vi "busy_wait_embed.vi"(4 "dialog_reference":refnum<vi>, 6 "knob_reference":refnum<vi>, 7 "caller":refnum<vi>, 8 "error in (no error)":errorcluster, 11 "configuration":T1={"dialog_text"="", "boolean_text_1"="", "boolean_text_2"="", "boolean_text_3"="", "inner_color"=16711680, "outer_color"=6618880, "wait_s"=nan, "error_status"=FALSE, "error_source"="", "error_details"="", "string []"=[], "custom_entry"=FALSE}) -> (0 "error out":errorcluster, 3 "failed/cancelled?":bool)   [LabVIEW 2015, in "lv-dialog-interfaces.lvlib"]
uses:
  lv-dialog-interfaces.lvlib
  lv-dialog/api/v1/public/_controls/configuration.ctl
  _controls/dialog_type.ctl
  _controls/hmi_references.ctl
  lv-dialog/api/v1/public/_controls/dialog_selection.ctl
  <vilib>/ptbypt/NI_PtbyPt.lvlib
  lv-dialog/api/v1/v1.lvlib
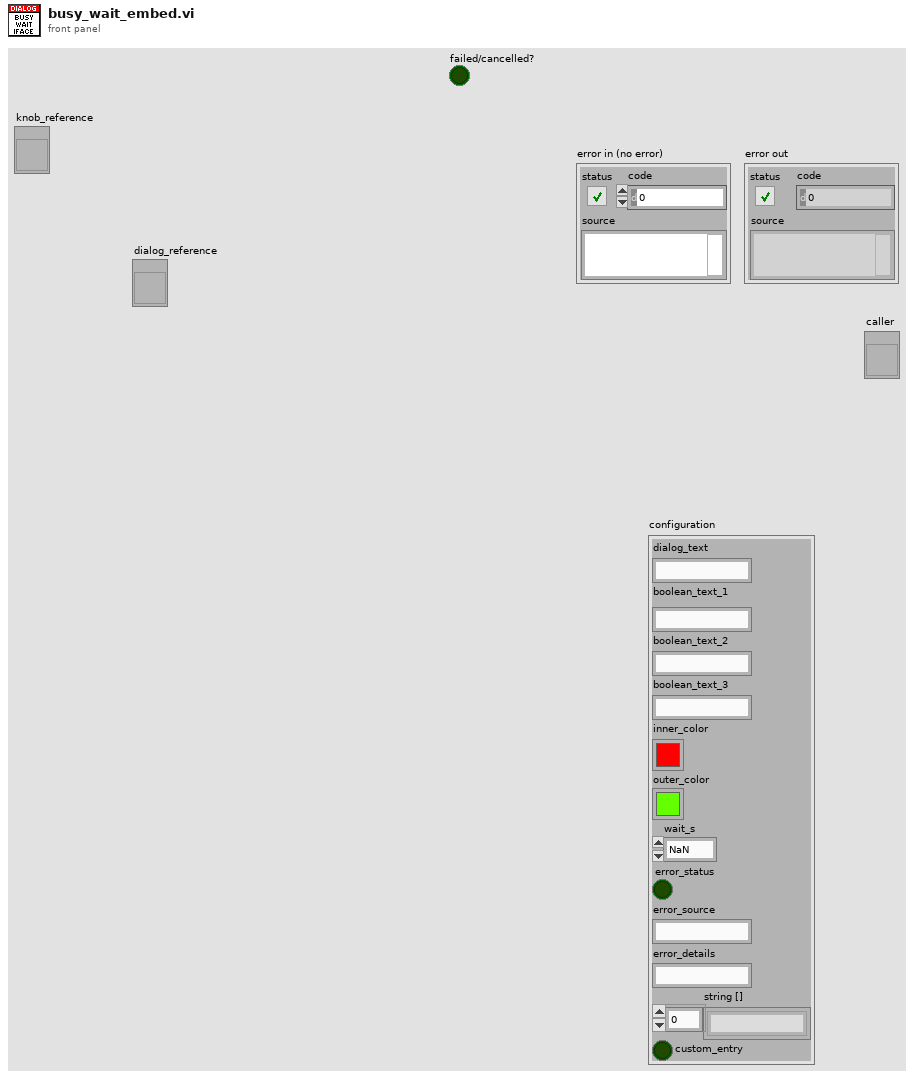
[diagram p1: front panel]
types:
  T1 = typedef "lv-dialog.lvlib/v1.lvlib/configuration.ctl" = cluster{"dialog_text":string, "boolean_text_1":string, "boolean_text_2":string, "boolean_text_3":string, "inner_color":u32, "outer_color":u32, "wait_s":dbl, "error_status":bool, "error_source":string, "error_details":string, "string []":string[], "custom_entry":bool}
  T2 = typedef "lv-dialog-interfaces.lvlib/dialog_type.ctl" = enum16{"null", "one_button", "two_button", "three_button", "confirmation", "busy_wait", "error", "busy_wait_embed", "combo_box", "data_entry_string", "data_entry_numeric"}
  T3 = typedef "lv-dialog-interfaces.lvlib/hmi_references.ctl" = cluster{"vi_reference":refnum<vi>, "caller":refnum<vi>, "dialog":refnum<vi>, "button_1":refnum<vi>, "button_2":refnum<vi>, "button_3":refnum<vi>, "busy":refnum<vi>, "error_glyph":refnum<vi>, "error_source":refnum<vi>, "error_text":refnum<vi>, "combo_box":refnum<vi>}
  T4 = typedef "lv-dialog.lvlib/v1.lvlib/dialog_selection.ctl" = enum16{"null", "panel_closed", "button_1", "button_2", "button_3", "cancelled"}
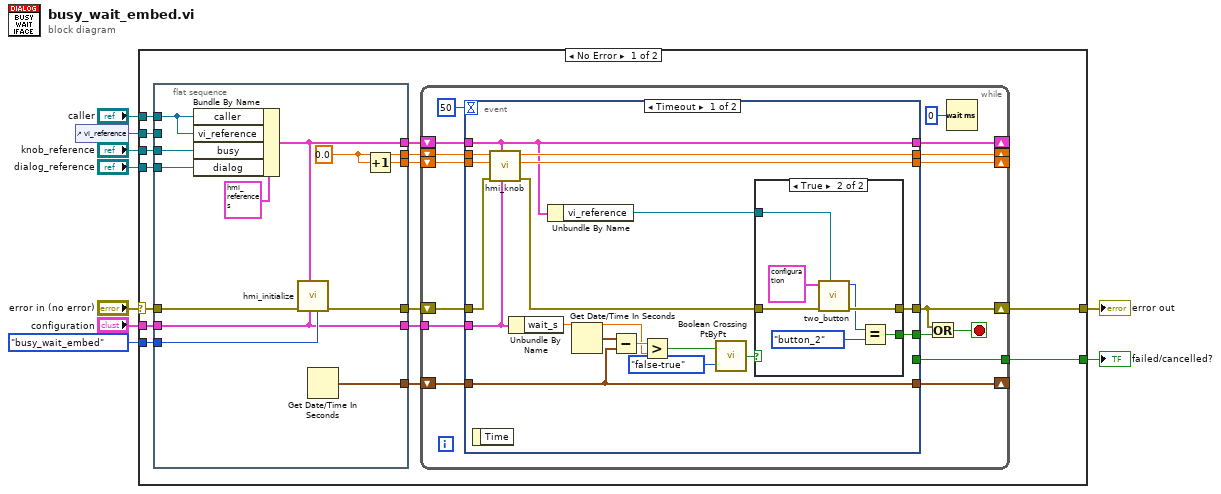
[diagram p0: block diagram]
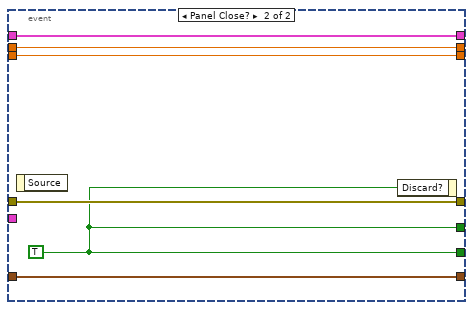
[diagram p3: hidden frame]
diagram:
  n1 = control-ref of="vi_reference"() -> (w1:refnum<vi>)
  n2 = case shown="No Error" "error in (no error)" {
    selector: "error in (no error)" -> [w24 w85]
    tunnel: [w23 _] -> w8
    tunnel: "caller" -> [w22 _]
    tunnel: "configuration" -> [w21 _]
    tunnel: dialog_type."busy_wait_embed" ("dialog_type") -> [w20 _]
    tunnel: [w10 w85] -> w4
    tunnel: "knob_reference" -> [w13 _]
    tunnel: "dialog_reference" -> [w12 _]
    tunnel: w1 -> [w11 _]
    frame No Error {
      n3 = flat-sequence {
        tunnel: [w36] -> w19
        tunnel: [w35] -> w18
        tunnel: [w29] -> w17
        tunnel: w24 -> [w34]
        tunnel: [w31] -> w16
        tunnel: [w30] -> w15
        tunnel: w21 -> [w28]
        tunnel: [w28] -> w14
        tunnel: w22 -> [w25]
        tunnel: w20 -> [w32]
        tunnel: w13 -> [w27]
        tunnel: w12 -> [w26]
        tunnel: w11 -> [_]
        frame #0 {
          w30 = 0.0
          n4 = Bundle By Name(cluster=T3 {"vi_reference"=refnum, "caller"=refnum, "dialog"=refnum, "button_1"=refnum, "button_2"=refnum, "button_3"=refnum, "busy"=refnum, "error_glyph"=refnum, "error_source"=refnum, "error_text"=refnum, "combo_box"=refnum} ("references"), "caller"=w25, "vi_reference"=w25, "busy"=w27, "dialog"=w26) -> (w29:T3)
          n5 = call "hmi_initialize.vi"("dialog_type"=w32, "configuration"=w28, "references"=w29, "error in (no error)"=w34) -> ("error out"=w31:errorcluster)  [unwired: 7 in]
          n6 = Get Date/Time In Seconds() -> (seconds since 1Jan1904=w35:timestamp)
          n7 = Increment(x=w30) -> (x+1=w36:dbl)
        }
      }
      n8 = while {
        shift-right: [w52] -> _
        shift-left: w15 -> [w49]
        shift-right: [w51] -> _
        shift-left: w19 -> [w50]
        shift-right: [w38] -> w10
        shift-left: w16 -> [w48]
        shift-right: [w44] -> _
        shift-left: w18 -> [w45]
        tunnel: [w43] -> w23
        tunnel: w14 -> [w42]
        shift-right: [w37] -> _
        shift-left: w17 -> [w41]
        stop <- w39 stop-if-true
        n9 = event shown="[0] Timeout" {
          selector: _ -> [_ _]
          dyn-events: _ -> [_ _]
          timeout: 50 -> [_ _]
          tunnel: [w60 w83] -> w52
          tunnel: [w61 w82] -> w51
          tunnel: w50 -> [w59 w82]
          tunnel: w49 -> [w58 w83]
          tunnel: w48 -> [w70 w84]
          tunnel: [w63 w84] -> w38
          tunnel: [w53 w81] -> w40
          tunnel: w45 -> [w68 w80]
          tunnel: [w68 w80] -> w44
          tunnel: [w53 w81] -> w43
          tunnel: w42 -> [w56 _]
          tunnel: w41 -> [w55 w79]
          tunnel: [w55 w79] -> w37
          event Timeout {
            n10 = event-data() -> ()  [unwired: 1 in, 1 out]
            n11 = call "hmi_knob.vi"("configuration"=w56, "hmi_references"=w55, "error in (no error)"=w70, "value_2 in"=w59, "value_1 in"=w58) -> ("error out"=w64:errorcluster, "value_2 out"=w61:dbl, "value_1 out"=w60:dbl)  [unwired: 4 in]
            n12 = Unbundle By Name(w56) -> ("wait_s"=w57:dbl)
            n13 = Unbundle By Name(w55) -> ("vi_reference"=w54:refnum<vi>)
            n14 = Get Date/Time In Seconds() -> (seconds since 1Jan1904=w69:timestamp)
            n15 = Subtract(x=w69, y=w68) -> (x-y=w67:dbl)
            n16 = Greater?(x=w67, y=w57) -> (0:w66:bool)
            n17 = call <vilib>:"Boolean Crossing PtByPt.vi"("direction"=enum16{"either", "false-true", "true-false"}."false-true", "input"=w66) -> ("crossing"=w62:bool)  [unwired: 1 in]
            n18 = case shown="True" w62 {
              tunnel: w64 -> [w71 w76]
              tunnel: [w71 w75] -> w63
              tunnel: [_ w77] -> w53
              tunnel: w54 -> [_ w74]
              frame False {
              }
              frame True {
                n19 = call "two_button.vi"("callee"=w74, "error in (no error)"=w76, "configuration"=T1 {"dialog_text"="Waiting process has not completed.", "boolean_text_1"="Wait", "boolean_text_2"="Continue", "boolean_text_3"="", "inner_color"=16711680, "outer_color"=6618880, "wait_s"=nan, "error_status"=FALSE, "error_source"="", "error_details"="", "string []"=[], "custom_entry"=FALSE} ("configuration 2")) -> ("error out"=w75:errorcluster, "dialog_selection"=w73:T4)  [unwired: 7 in]
                n20 = Equal?(x=w73, y=dialog_selection."button_2" ("x")) -> (x = y?=w77:bool)
              }
            }
          }
          event Panel Close? {
            w81 = TRUE
            n21 = event-data() -> ()  [unwired: 1 in, 1 out]
            n22 = event-data("Discard?"=w81) -> ()  [unwired: 1 in, 1 out]
          }
        }
        n23 = Or(x=w38, y=w40) -> (x .or. y?=w39:bool)
        n24 = Wait (ms)(milliseconds to wait=u32 0) -> ()  [unwired: 1 out]
      }
    }
    frame Error {
    }
  }
  "error out" <- w4
  "failed/cancelled?" <- w8
